vi "Release Helper Loop Q DVR.vi"(10 "Helper Loop Q DVR":refnum<data-value>) -> (0 "error out":errorcluster)   [LabVIEW 2021, in "Helper Loop.lvclass"]
uses:
  Helper Loop.lvclass
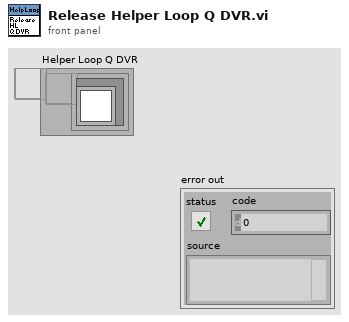
[diagram p1: front panel]
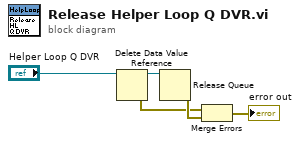
[diagram p0: block diagram]
diagram:
  n1 = Delete Data Value Reference(data value reference="Helper Loop Q DVR") -> (data value=w5:refnum<queue>, error out=w3:errorcluster)  [unwired: 1 in]
  n2 = Release Queue(queue=w5) -> (error out=w4:errorcluster)  [unwired: 2 in, 2 out]
  n3 = Merge Errors(w3, w4) -> (→"error out":errorcluster)
